vi "NI Scope Lockin.vi"() -> ()   [LabVIEW 2016]
uses:
  <instrlib>/niScope/Controls/niScope trigger source digital.ctl
  <instrlib>/niScope/Configure/Trigger/niScope Configure Trigger Digital.vi
  <instrlib>/niScope/Acquire/Fetch/niScope Multi Fetch Binary 16.vi
panel:
  out "Fetch:Points Done":dbl
  in  "Ext clock":bool=TRUE
  in  "Group name":string="p"
  in  "Channel names":string[](array[string])
  in  "Plot":bool
  in  "Save":bool
  in  "Route":bool
  in  "destination terminal":tag="/5105-PXI/PXI_Trig0"
  in  "source terminal":tag="/6133/PFI0"
  out "size(s)":i32[](array[numeric])
  out "x-y":i32
  out "Waveform Graph":i16[][](graph)
  out "acquisition status":i32
  in  "numSamples per read":i32=100000 caption="numSamples to fetch" format="%.0p"
  in  "trigger source":T1="VAL_RTSI_0"
  in  "min record length":i32=1000000 format="%.0p"
  in  "reference position":dbl=50.0 format="%.1f"
  in  "min sample rate":dbl=18943964.8 caption="sample rate" format="%^.2e"
  in  "channels":string="0"
  in  "reset device":bool=TRUE
  in  "resource name":refnum<k15>="5105-PCI"
  # "VAL_NO_SOURCE\nVAL_PFI_1"
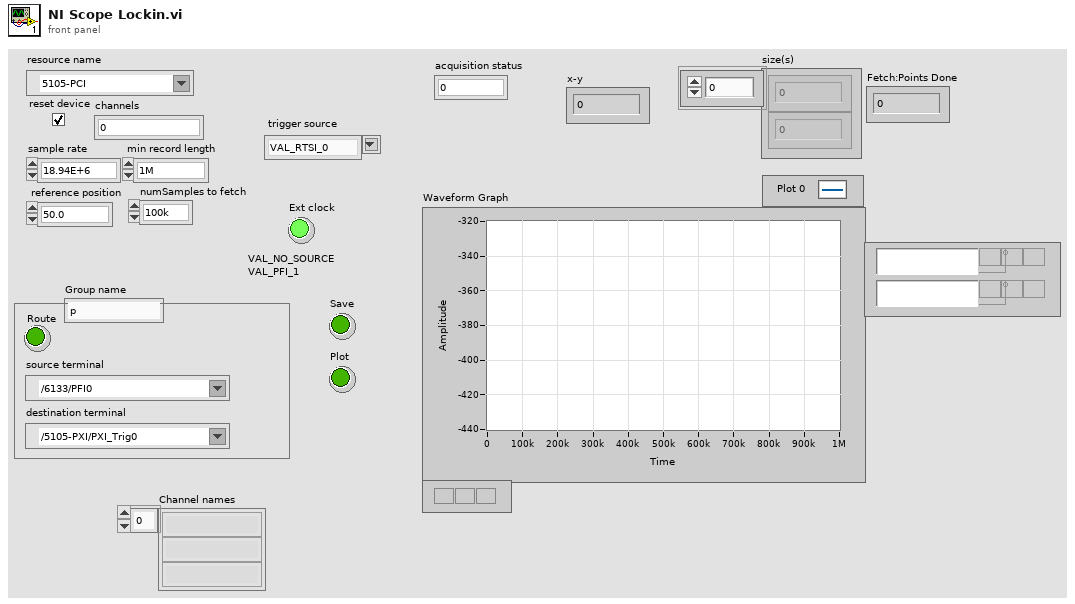
[diagram p1: front panel]
types:
  T1 = typedef "niScope trigger source digital.ctl" = string
  T2 = enum16{"open", "open or create", "create or replace", "create", "open (read-only)"}
  T3 = cluster{"actualSamples":i32, "absoluteInitialX":dbl, "relativeInitialX":dbl, "xIncrement":dbl, "offset":dbl, "gain":dbl, "reserved1":dbl, "reserved2":dbl}[]
  T4 = cluster{"actualSamples":i32, "absoluteInitialX":dbl, "relativeInitialX":dbl, "xIncrement":dbl, "offset":dbl, "gain":dbl, "reserved1":dbl, "reserved2":dbl}
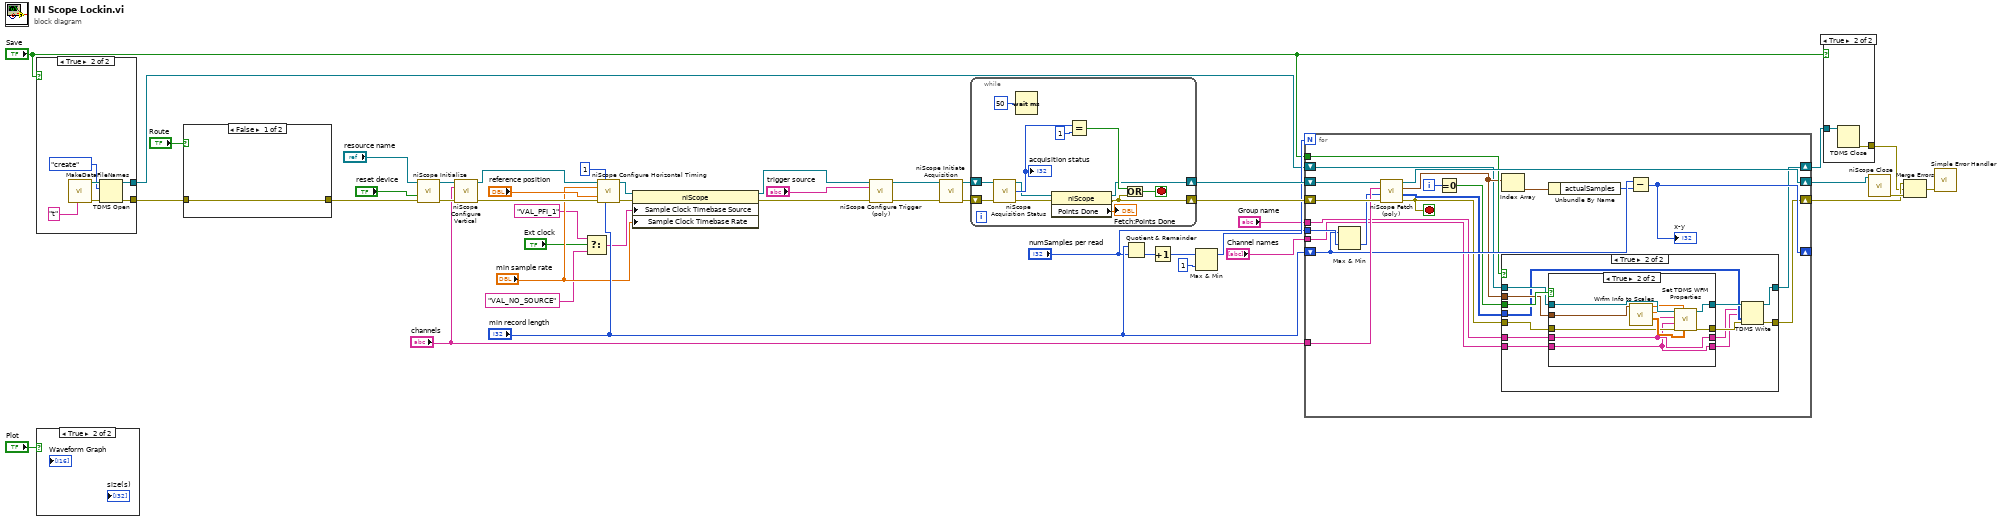
[diagram p0: block diagram]
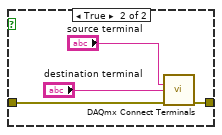
[diagram p5: hidden frame]
diagram:
  n1 = case shown="True" "Save" {
    tunnel: [_ w47] -> w13
    tunnel: [_ w46] -> w12
    frame False {
    }
    frame True {
      n2 = call "MakeDataFileNames.vi"("File Prefix"="t") -> ("Error Out"=w50:errorcluster, "Data File  Path"=w49:path)  [unwired: 7 in, 2 out]
      n3 = TDMS Open(8:w50, 10:T2."create" ("operation (0:open)"), 11:w49) -> (0:w46:errorcluster, 3:w47:refnum<k34>)  [unwired: 4 in]
    }
  }
  n4 = case shown="True" "Plot" {
    frame False {
    }
    frame True {
    }
  }
  n5 = case shown="False" "Route" {
    tunnel: [w52 w54] -> w15
    tunnel: w12 -> [w52 w53]
    frame False {
    }
    frame True {
      n6 = call <vilib>:"DAQmx Connect Terminals.vi"("source terminal"="source terminal", "destination terminal"="destination terminal", "error in"=w53) -> ("error out"=w54:errorcluster)  [unwired: 12 in]
    }
  }
  n7 = call <instrlib>:"niScope Initialize.vi"("resource name"="resource name", "reset device"="reset device", "error in"=w15) -> ("instrument handle"=w43:refnum<k15>, "error out"=w42:errorcluster)  [unwired: 11 in]
  n8 = call <instrlib>:"niScope Configure Vertical.vi"("instrument handle"=w43, "channels"="channels", "error in"=w42) -> ("instrument handle out"=w41:refnum<k15>, "error out"=w40:errorcluster)  [unwired: 11 in]
  n9 = Select(t="VAL_PFI_1", s="Ext clock", f="VAL_NO_SOURCE") -> (s? t:f=w1:string)
  n10 = call <instrlib>:"niScope Configure Horizontal Timing.vi"("instrument handle"=w41, "number of records"=1, "min sample rate"="min sample rate", "reference position"="reference position", "error in"=w40, "min record length"="min record length") -> ("instrument handle out"=w38:refnum<k15>, "error out"=w35:errorcluster)  [unwired: 8 in]
  n11 = property class="niScope"(reference=w38, error in=w35, "Sample Clock Timebase Source"=w1, "Sample Clock Timebase Rate"="min sample rate") -> (reference out=w37:refnum<k15>, error out=w36:errorcluster)
  n12 = call-poly <instrlib>:"niScope Configure Trigger (poly).vi"("instrument handle"=w37, "trigger source"="trigger source", "error in"=w36) -> ("instrument handle out"=w31:refnum<k15>, "error out"=w32:errorcluster)  [unwired: 4 in, 7 out]
  n13 = call <instrlib>:"niScope Initiate Acquisition.vi"("instrument handle"=w31, "error in"=w32) -> ("instrument handle out"=w30:refnum<k15>, "error out"=w29:errorcluster)  [unwired: 12 in]
  n14 = while {
    shift-right: [w60] -> w27
    shift-left: w29 -> [w67]
    shift-right: [w58] -> w28
    shift-left: w30 -> [w68]
    stop <- w62 stop-if-true
    n15 = call <instrlib>:"niScope Acquisition Status.vi"("instrument handle"=w68, "error in"=w67) -> ("instrument handle out"=w59:refnum<k15>, "acquisition status"=w64:i32, "error out"=w61:errorcluster)  [unwired: 11 out]
    "acquisition status" <- w64
    n16 = Wait (ms)(milliseconds to wait=u32 50) -> ()  [unwired: 1 out]
    n17 = property class="niScope"(reference=w59, error in=w61) -> (reference out=w58:refnum<k15>, error out=w60:errorcluster, "Points Done"=→"Fetch:Points Done":dbl)
    n18 = Equal?(x=w64, y=1) -> (x = y?=w65:bool)
    n19 = Or(x=w65, y=w60) -> (x .or. y?=w62:bool)
  }
  n20 = Quotient & Remainder(x="min record length", y="numSamples per read") -> (floor(x/y)=w25:i32)  [unwired: 1 out]
  n21 = Increment(x=w25) -> (x+1=w24:i32)
  n22 = Max & Min(x=w24, y=1) -> (max(x,y)=w21:i32)  [unwired: 1 out]
  n23 = for {
    N: w21 -> [_]
    tunnel: "channels" -> [w87]
    tunnel: "numSamples per read" -> [w83]
    shift-right: [w70] -> w6
    shift-left: w27 -> [w88]
    shift-right: [w86] -> w23
    shift-left: w28 -> [w89]
    shift-right: [w84] -> _
    shift-left: "min record length" -> [w82]
    tunnel: "Save" -> [w79]
    tunnel: "Channel names" -> [w74]
    tunnel: "Group name" -> [w73]
    shift-right: [w69] -> w9
    shift-left: w13 -> [w75]
    i -> [w78]
    stop <- w72 stop-if-true
    n24 = Max & Min(x=w82, y=w83) -> (min(x,y)=w81:i32)  [unwired: 1 out]
    n25 = call-poly <instrlib>:"niScope Fetch (poly).vi"("error in"=w88, "numSamples"=w81, "channels"=w87, "instrument handle"=w89) -> ("error out"=w72:errorcluster, "wfm"=w71:i16[][], "wfm info"=w76:T3, "instrument handle out"=w86:refnum<k15>)  [unwired: 4 in]
    n26 = Equal To 0?(x=w78) -> (x = 0?=w77:bool)
    n27 = Index Array(array=w76) -> (element=w85:T4)  [unwired: 1 in]
    n28 = case shown="True" w79 {
      tunnel: w77 -> [_ w104]
      tunnel: w76 -> [_ w103]
      tunnel: w75 -> [w90 w102]
      tunnel: w74 -> [_ w101]
      tunnel: w73 -> [_ w100]
      tunnel: w72 -> [w91 w99]
      tunnel: w71 -> [_ w96]
      tunnel: [w91 w93] -> w70
      tunnel: [w90 w92] -> w69
      frame False {
      }
      frame True {
        n29 = case shown="True" w104 {
          tunnel: w103 -> [_ w118]
          tunnel: w102 -> [w107 w117]
          tunnel: w101 -> [w106 w109]
          tunnel: w100 -> [w105 w110]
          tunnel: w99 -> [w108 w113]
          tunnel: [w108 w112] -> w98
          tunnel: [w107 w111] -> w97
          tunnel: [w106 w109] -> w95
          tunnel: [w105 w110] -> w94
          frame False {
          }
          frame True {
            n30 = call "Wrfm Info to Scales.vi"("wfm info"=w118) -> ("Scaling coefficients"=w116:dbl[][], "dt"=w114:dbl, "t0"=w115:dbl)  [unwired: 8 in]
            n31 = call "Set TDMS WFM Properties.vi"("dt"=w114, "Scaling coefficients"=w116, "t0"=w115, "error in (no error)"=w113, "Channel names"=w109, "Group name"=w110, "tdms file"=w117) -> ("error out"=w112:errorcluster, "tdms file out"=w111:refnum<k34>)  [unwired: 3 in]
          }
        }
        n32 = TDMS Write(0:w97, 5:w94, 7:w95, 9:w96, 11:w98) -> (4:w92:refnum<k34>, 15:w93:errorcluster)  [unwired: 1 in, 2 out]
      }
    }
    n33 = Unbundle By Name(w85) -> ("actualSamples"=w80:i32)
    n34 = Subtract(x=w82, y=w80) -> (x-y=w84:i32)
    "x-y" <- w84
  }
  n35 = case shown="True" "Save" {
    tunnel: w9 -> [_ w120]
    tunnel: [_ w119] -> w5
    frame False {
    }
    frame True {
      n36 = TDMS Close(11:w120) -> (0:w119:errorcluster)  [unwired: 1 in, 1 out]
    }
  }
  n37 = call <instrlib>:"niScope Close.vi"("instrument handle"=w23) -> ("error out"=w22:errorcluster)  [unwired: 14 in]
  n38 = Merge Errors(w6, w5, w22) -> (w7:errorcluster)
  n39 = call <vilib>:"Simple Error Handler.vi"("error in (no error)"=w7) -> ()  [unwired: 4 in, 5 out]
